vi "IAmGLF-SendToStandaloneProcess.vi"(8 "error in (no error)":errorcluster, 10 "Class Return Notifier":refnum<notifier>, 11 "Engine in":refnum<class "Engine.lvclass">) -> (0 "error out":errorcluster, 3 "Engine out":refnum<class "Engine.lvclass">)   [LabVIEW 2024, in "GLF.lvlib" / "Engine.lvclass"]
doc: "<B>Summary</B>\nUsed to send <B>IAmGLF</B> along with <B>Data</B> to a standalone entity in order for it to create the class internal DVR.\n\n<B>Details</B>\nThis is done that way because LabVIEW automatically releases references created by VIs (or their callers) that are no longer running. So we must rely on an another asych process to be sure the DVR is not deleted."
uses:
  Engine.lvclass
  IAmGLF/IAmGLF.lvclass
  Core.vi
  Engine.lvclass/Engine.ctl
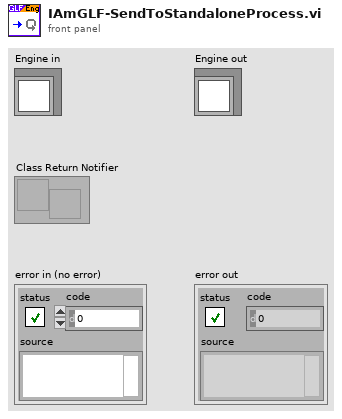
[diagram p1: front panel]
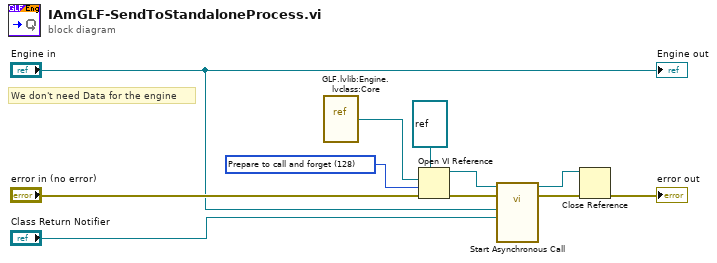
[diagram p0: block diagram]
diagram:
  w5 = 128 items=["Record modifications"=1, "Open templates for editing"=2, "Prompt user to save"=4, "Prepare for reentrant run"=8, "Prompt to find missing subVIs"=16, "Hide loading dialog box"=32, "Enable simultaneous calls"=64, "Prepare to call and forget"=128, "Simultaneous call and forget"=192, "Prepare to call and collect"=256, "Simultaneous call and collect"=320]
  # "We don't need Data for the engine"
  n1 = vi-ref "GLF.lvlib:Engine.lvclass:Core.vi"() -> (w7:refnum<vi>)
  n2 = Open VI Reference(type specifier VI Refnum (for type only)=refnum<vi> refnum, vi path=w7, options=w5, error in (no error)="error in (no error)") -> (vi reference=w9:refnum<vi>, error out=w11:errorcluster)  [unwired: 2 in]
  n3 = call-by-ref "Start Asynchronous Call"(reference=w9, error in=w11, "Class Return Notifier"="Class Return Notifier", "Engine in"="Engine in") -> (reference out=w8:refnum<vi>, error out=w10:errorcluster)  [unwired: 10 in]
  n4 = Close Reference(reference=w8, error in (no error)=w10) -> (error out=→"error out":errorcluster)
  "Engine out" <- "Engine in"
